vi "create JSONPacket.vi"(8 "error in (no error)":errorcluster, 10 "Variant":variant, 11 "JSONPacket in":refnum<class "JSONPacket.lvclass">) -> (0 "error out":errorcluster, 3 "JSONPacket out":refnum<class "JSONPacket.lvclass">)   [LabVIEW 2019, in "JSONPacket.lvclass"]
uses:
  JSONPacket.lvclass
  C:/projects/labview_multiplayer_snake_personal/Main Codeline/Software/Code/Shared/TCPPacket/TCPPacket.lvclass
  TCPPacket/TCPHeader ContentType STYP.ctl
  TCPPacket/TCPHeader ContentEncoding STYP.ctl
  JSONPacket.lvclass/JSONPacket.ctl
  TCPPacket/TCPPacket.lvclass
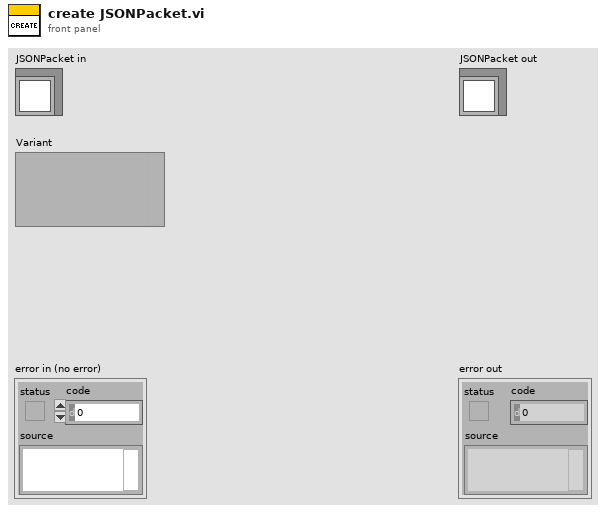
[diagram p1: front panel]
types:
  T1 = typedef "TCPPacket.lvclass/TCPHeader ContentEncoding STYP.ctl" = enum16{"binary", "utf-8", "latin-1"}
  T2 = typedef "TCPPacket.lvclass/TCPHeader ContentType STYP.ctl" = enum16{"text/json", "binary/application"}
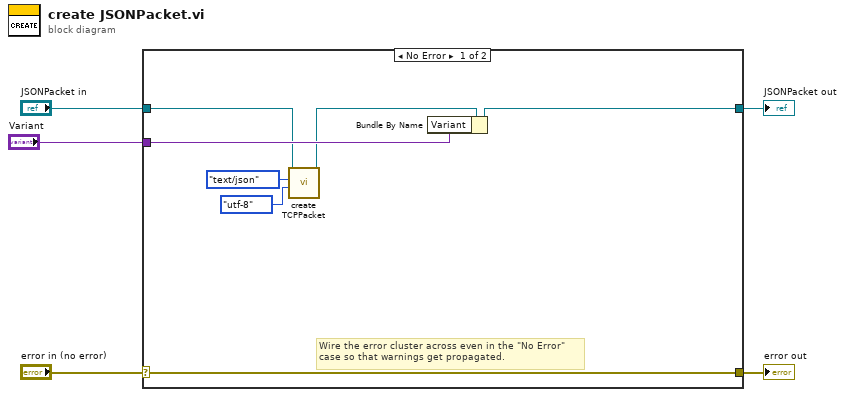
[diagram p0: block diagram]
diagram:
  n1 = case shown="No Error" "error in (no error)" {
    selector: "error in (no error)" -> [w12 w14]
    tunnel: [w12 w14] -> w4
    tunnel: [w11 w13] -> w2
    tunnel: "JSONPacket in" -> [w8 w13]
    tunnel: "Variant" -> [w10 _]
    frame No Error {
      # "Wire the error cluster across even in the \"No Error\"\ncase so that warnings get propagated."
      n2 = call "create TCPPacket.vi"("Encoding"=TCPHeader_ContentEncoding_STYP."utf-8", "Content Type"=TCPHeader_ContentType_STYP."text/json", "TCPPacket in"=w8) -> ("TCPPacket out"=w9:refnum<class "JSONPacket.lvclass">)  [unwired: 7 in, 1 out]
      n3 = Bundle By Name(cluster=w9, "Variant"=w10) -> (w11:refnum<class "JSONPacket.lvclass">)
    }
    frame Error {
    }
  }
  "error out" <- w4
  "JSONPacket out" <- w2
